vi "Tools_KeyedArray Convert from XML Children.vi"(8 "error in (no error)":errorcluster, 11 "KA String":string="<DB_Connection>c:\\temp</DB_Connection>") -> (0 "error out":errorcluster, 3 "keyed array":T1)   [LabVIEW 2012]
uses:
  Tools_KeyedArray KeyedArray.ctl
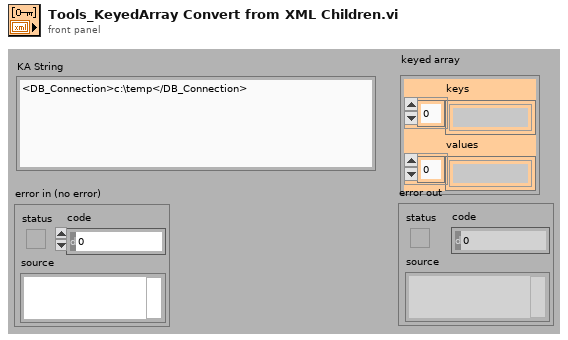
[diagram p1: front panel]
types:
  T1 = typedef "Tools_KeyedArray KeyedArray.ctl" = cluster{"keys":string[], "values":string[]}
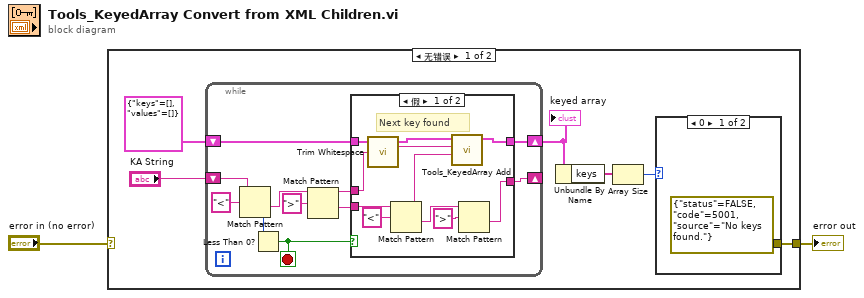
[diagram p0: block diagram]
diagram:
  n1 = case shown="无错误" "error in (no error)" {
    selector: "error in (no error)" -> [_ w33]
    tunnel: [w3 w33] -> w1
    frame No Error {
      n2 = while {
        shift-right: [w14] -> _
        shift-left: "KA String" -> [w20]
        shift-right: [w15] -> w6
        shift-left: T1 {"keys"=[], "values"=[]} ("keyed array") -> [w16]
        stop <- w17 stop-if-true
        n3 = Match Pattern(string=w20, regular expression="<") -> (after substring=w13:string, offset past match=w18:i32)  [unwired: 3 out]
        n4 = Less Than 0?(x=w18) -> (x < 0?=w17:bool)
        n5 = Match Pattern(string=w13, regular expression=">") -> (before substring=w11:string, after substring=w10:string)  [unwired: 3 out]
        n6 = case shown="假" w17 {
          tunnel: w11 -> [w30 _]
          tunnel: w16 -> [w29 w32]
          tunnel: [w28 w32] -> w15
          tunnel: w10 -> [w21 w31]
          tunnel: [w23 w31] -> w14
          frame False {
            # "Next key found"
            n7 = call <vilib>:"Trim Whitespace.vi"("string"=w30) -> ("trimmed string"=w27:string)  [unwired: 1 in]
            n8 = Match Pattern(string=w21, regular expression="<") -> (before substring=w22:string, after substring=w25:string)  [unwired: 3 out]
            n9 = call "Tools_KeyedArray Add.vi"("value"=w22, "key"=w27, "array in"=w29) -> ("array out"=w28:T1)  [unwired: 1 in, 3 out]
            n10 = Match Pattern(string=w25, regular expression=">") -> (after substring=w23:string)  [unwired: 4 out]
          }
          frame True {
            # "No key found"
          }
        }
      }
      "keyed array" <- w6
      n11 = Unbundle By Name(w6) -> ("keys"=w5:string[])
      n12 = Array Size(array=w5) -> (size(s)=w4:i32)
      n13 = case shown="0" w4 {
        tunnel: [errorcluster {"status"=FALSE, "code"=5001, "source"="No keys found."} ("error IO") _] -> w3
        frame 0 {
        }
        frame 1, Default {
        }
      }
    }
    frame Error {
    }
  }
  "error out" <- w1
